vi "Initialize.vi"(7 "CD Name":string, 8 "error in":errorcluster, 9 "Compiled Settings":variant, 10 "CDAPI in":refnum<class "CustomDeviceAPI.lvclass">, 11 "CD in":refnum<class "Template.lvclass">) -> (0 "error out":errorcluster, 3 "CD out":refnum<class "Template.lvclass">)   [LabVIEW 2026, in "Template Plugin.lvlib" / "Template.lvclass"]
uses:
  Template.lvclass
  Template.lvclass/Template.ctl
  Types/TargetSettings.ctl
  SubVIs/Get Input Channel Group.vi
  SubVIs/Get Output Channel Group.vi
  <userlib>/CustomDeviceInterfaces_v1.lvlibp/custom-device-express-framework/Source/Custom Device Interfaces/CustomDeviceAPI/CustomDeviceAPI.lvclass
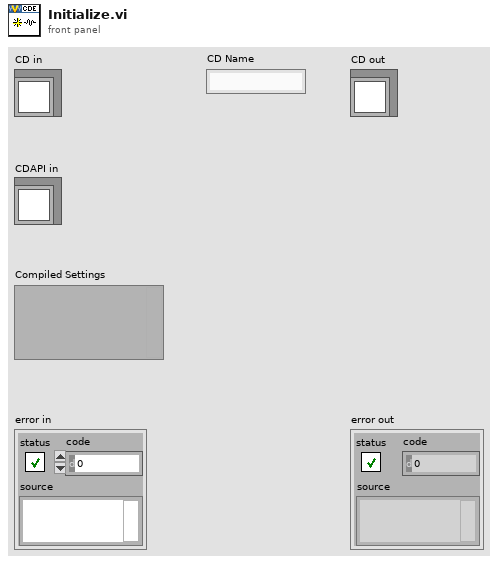
[diagram p1: front panel]
types:
  T1 = typedef "Template Plugin.lvlib/Template.lvclass/TargetSettings.ctl" = cluster{"Name":string}
  T2 = cluster{"Read":cluster{"Refs":cluster{"Data Reference":i32, "Offset":u64, "Length":u64}[], "Values":dbl[]}[], "Write":cluster{"Refs":cluster{"Data Reference":i32, "Offset":u64, "Length":u64}[], "Values":dbl[]}[], "ReadWrite":cluster{"Refs":i32[], "Values":dbl[], "Reset Values":dbl[]}[], "LUT":variant}
  T3 = cluster{"Refs":cluster{"Data Reference":i32, "Offset":u64, "Length":u64}[], "Values":dbl[]}
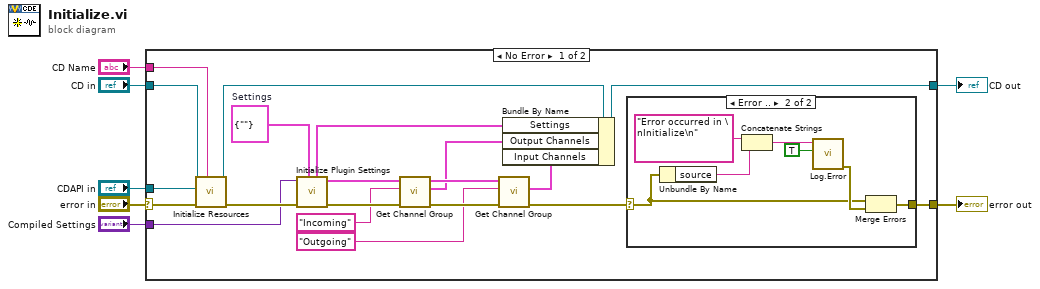
[diagram p0: block diagram]
diagram:
  n1 = case shown="No Error" "error in" {
    selector: "error in" -> [w27 w37]
    tunnel: "CD in" -> [w23 w36]
    tunnel: "CDAPI in" -> [w22 _]
    tunnel: [w21 w36] -> w3
    tunnel: [w8 w37] -> w6
    tunnel: "Compiled Settings" -> [w19 _]
    tunnel: "CD Name" -> [w25 _]
    frame No Error {
      w18 = T1 {"Name"=""}  # Settings
      n2 = call "Initialize Resources.vi"("CD Name"=w25, "error in"=w27, "CDAPI in"=w22, "Template in"=w23) -> ("error out"=w26:errorcluster, "Template out"=w24:refnum<class "Template.lvclass">)  [unwired: 6 in]
      n3 = call "Initialize Plugin Settings.vi"("Plugin Engine Settings in"=w18, "error in"=w26, "Compiled Settings"=w19) -> ("error out"=w20:errorcluster, "Channel Refs"=w16:T2, "Plugin Engine Settings out"=w17:T1)  [unwired: 6 in]
      n4 = call-poly "Get Channel Group.vi"("error in"=w20, "Group Name"="Incoming", "Channel Refs"=w16) -> ("error out"=w14:errorcluster, "Channel Group"=w11:T3, "Channel Refs"=w13:T2)  [unwired: 6 in]
      n5 = call-poly "Get Channel Group.vi"("error in"=w14, "Group Name"="Outgoing", "Channel Refs"=w13) -> ("error out"=w9:errorcluster, "Channel Group"=w10:T3)  [unwired: 6 in, 1 out]
      n6 = Bundle By Name(cluster=w24, "Settings"=w17, "Output Channels"=w11, "Input Channels"=w10) -> (w21:refnum<class "Template.lvclass">)
      n7 = case shown="Error .." w9 {
        selector: w9 -> [w28 w30]
        tunnel: [w28 w29] -> w8
        frame No Error {
        }
        frame Error {
          n8 = Unbundle By Name(w30) -> ("source"=w34:string)
          n9 = Concatenate Strings("Error occurred in \nInitialize\n" ("string"), w34) -> (w32:string)
          n10 = call "Log.Error.vi"("Add to log file? (F)"=TRUE, "Message"=w32) -> ("error out"=w31:errorcluster)  [unwired: 9 in]
          n11 = Merge Errors(w30, w31) -> (w29:errorcluster)
        }
      }
    }
    frame Error {
    }
  }
  "error out" <- w6
  "CD out" <- w3
